vi "UMLEditor ScriptTaskUpdateDiagram.vi"(0 "Folder/LLB-Path":path, 1 "AggregateClassPaths":path[](array[path]), 2 "BaseClass Folder/LLB-Path":path, 5 "error in (no error)":errorcluster, 6 "AggregateClassNames":string[](array[string])) -> (19 "error out":errorcluster)   [LabVIEW 2016]
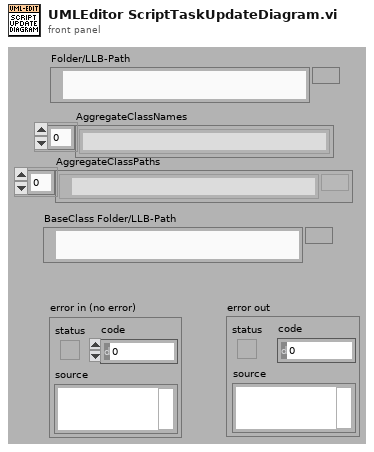
[diagram p1: front panel]
types:
  T1 = cluster{"CreateRef":refnum<vi>, "CreatePath":path, "CreateDiagram":refnum<vi>, "CalledCreatePaths":path[], "AggCreatePaths":path[], "DestroyRef":refnum<vi>, "DestroyPath":path, "DestroyDiagram":refnum<vi>, "CalledDestroyPaths":path[], "AggDestroyPaths":path[]}
  T2 = enum16{"NormalSubVis", "LV-Internal VIs", "All VIs", "All Functions"}
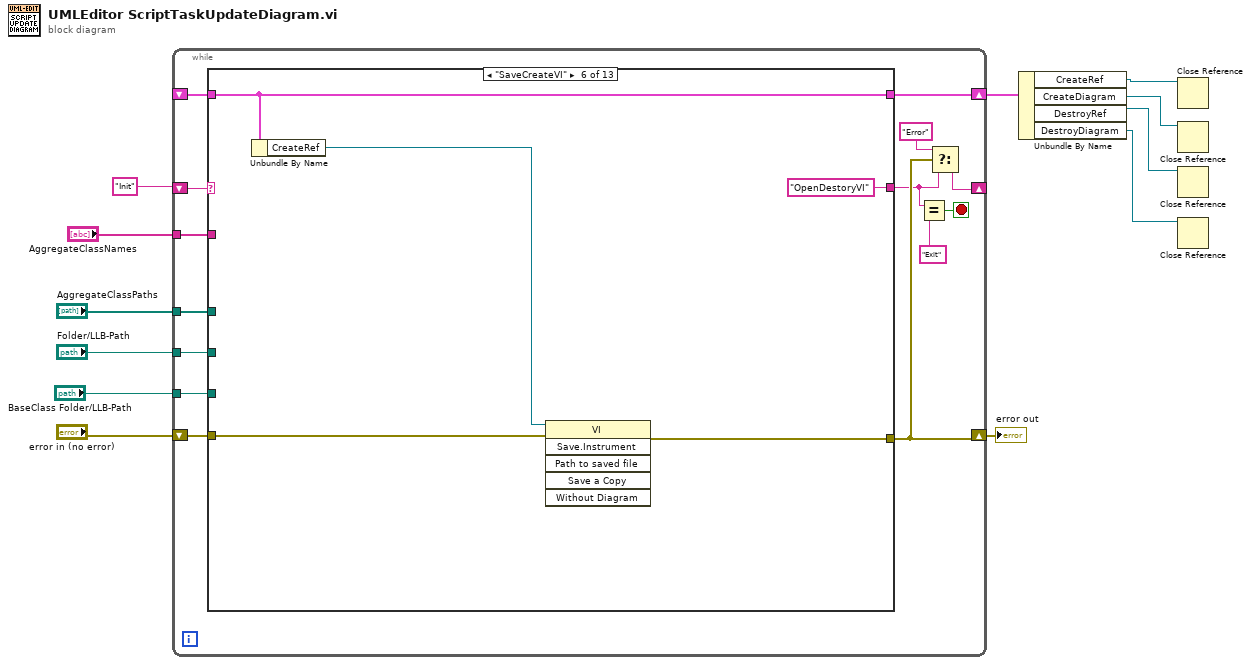
[diagram p0: block diagram]
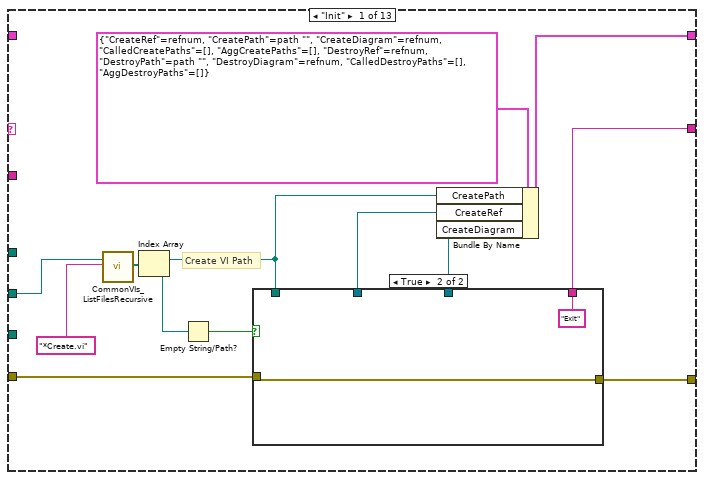
[diagram p2: hidden frame]
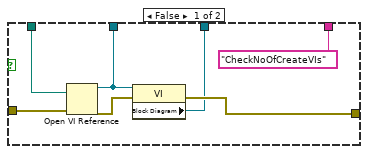
[diagram p3: hidden frame]
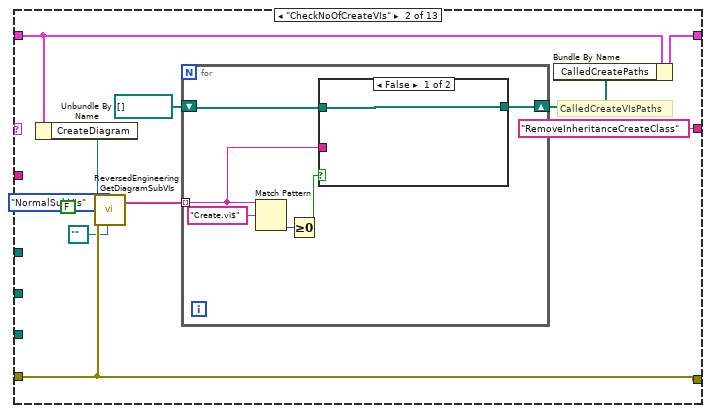
[diagram p4: hidden frame]
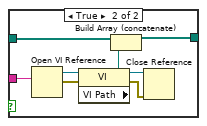
[diagram p5: hidden frame]
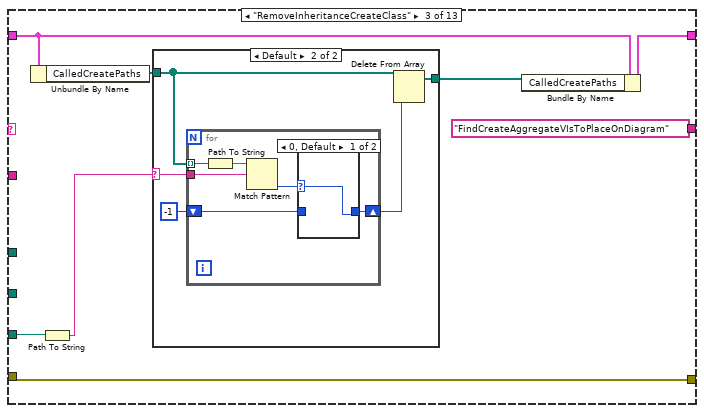
[diagram p6: hidden frame]
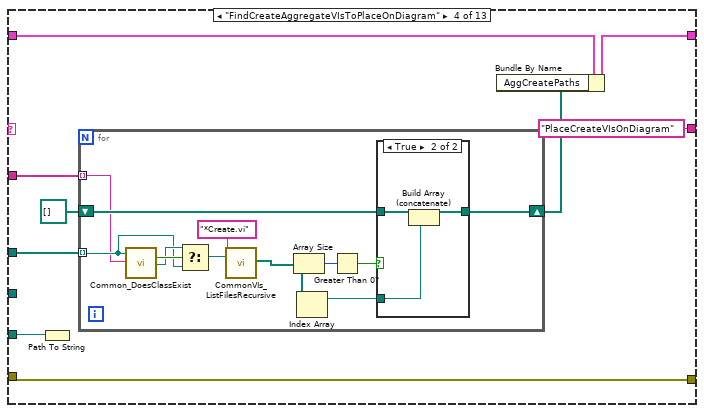
[diagram p9: hidden frame]
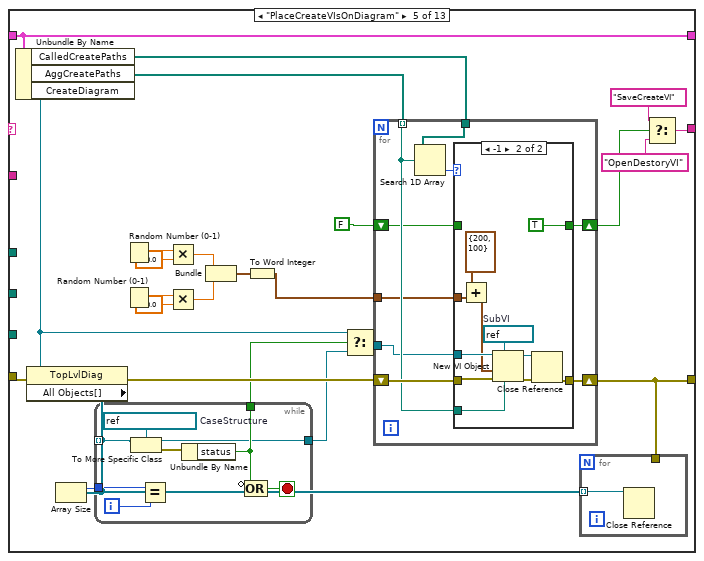
[diagram p11: hidden frame]
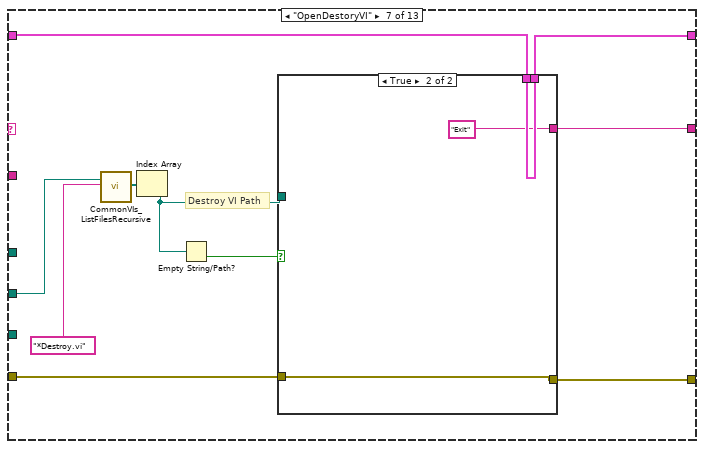
[diagram p13: hidden frame]
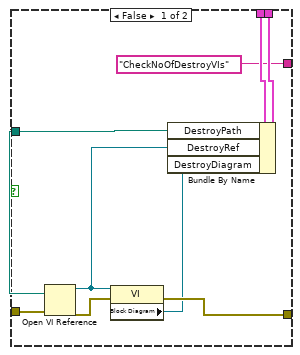
[diagram p14: hidden frame]
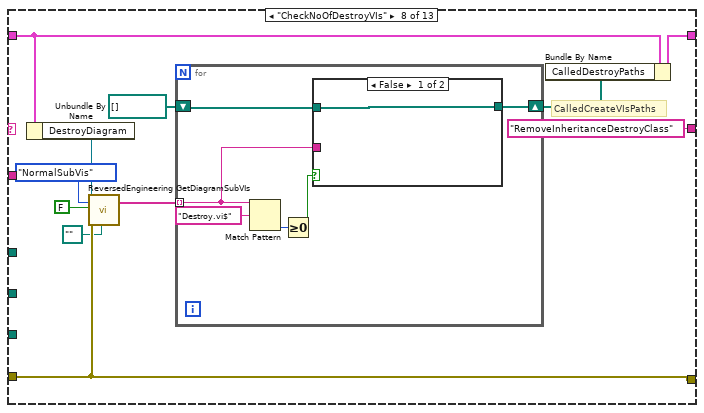
[diagram p15: hidden frame]
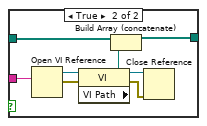
[diagram p16: hidden frame]
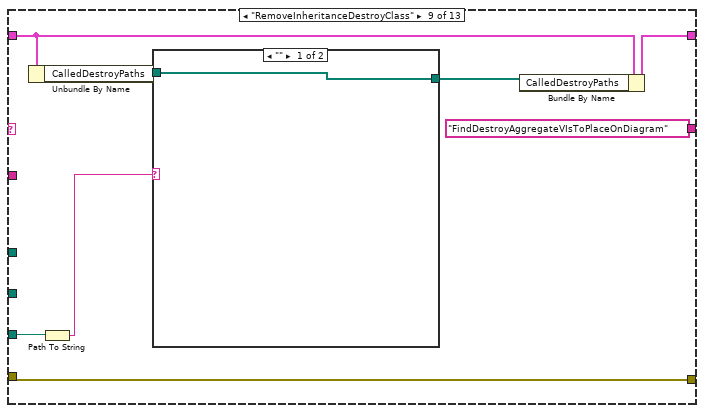
[diagram p17: hidden frame]
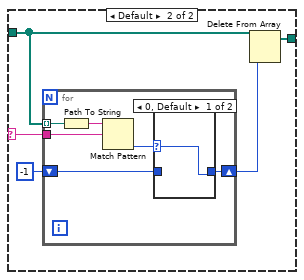
[diagram p18: hidden frame]
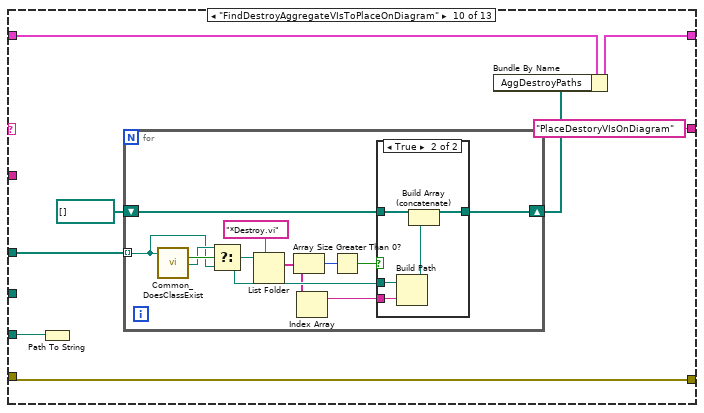
[diagram p20: hidden frame]
diagram:
  n1 = while {
    shift-right: [w23] -> _
    shift-left: "Init" -> [w26]
    shift-right: [w24] -> w9
    shift-left: "error in (no error)" -> [w25]
    shift-right: [w18] -> w11
    shift-left: _ -> [w17]
    tunnel: "Folder/LLB-Path" -> [w16]
    tunnel: "BaseClass Folder/LLB-Path" -> [w15]
    tunnel: "AggregateClassPaths" -> [w14]
    tunnel: "AggregateClassNames" -> [w13]
    stop <- w19 stop-if-true
    n2 = case shown="\"SaveCreateVI\"" w26 {
      selector: w26 -> [_ _ _ _ _ _ _ _ _ _ _ _ w340]
      tunnel: w25 -> [w38 w51 w76 w101 w141 w180 w191 w207 w232 w256 w297 w336 w339]
      tunnel: [w34 w51 w76 w101 w129 w178 w189 w207 w232 w256 w285 w334 w339] -> w24
      tunnel: [w27 "RemoveInheritanceCreateClass" "FindCreateAggregateVIsToPlaceOnDiagram" "PlaceCreateVIsOnDiagram" w133 "OpenDestoryVI" w182 "RemoveInheritanceDestroyClass" "FindDestroyAggregateVIsToPlaceOnDiagram" "PlaceDestoryVIsOnDiagram" w289 "Exit" "Exit"] -> w21
      tunnel: [w36 w54 w80 w103 w144 w177 w190 w210 w236 w258 w300 w333 w341] -> w18
      tunnel: w17 -> [_ w55 w81 w104 w144 w177 w188 w211 w237 w259 w300 w333 w341]
      tunnel: w16 -> [w32 _ _ _ _ _ w186 _ _ _ _ _ _]
      tunnel: w15 -> [_ _ w79 w102 _ _ _ _ w235 w257 _ _ _]
      tunnel: w14 -> [_ _ _ w99 _ _ _ _ _ w254 _ _ _]
      tunnel: w13 -> [_ _ _ w96 _ _ _ _ _ _ _ _ _]
      frame "Init" {
        # "Create VI Path"
        n3 = call <resource>:"CommonVIs_ListFilesRecursive.vi"("directory path"=w32, "FileSearchPattern"="*Create.vi" ("pattern")) -> ("Files"=w30:path[])  [unwired: 4 in, 13 out]
        n4 = Index Array(array=w30) -> (element=w29:path)  [unwired: 1 in]
        n5 = Empty String/Path?(string/path=w29) -> (empty?=w28:bool)
        n6 = case shown="True" w28 {
          tunnel: w38 -> [w45 w47]
          tunnel: w29 -> [w44 _]
          tunnel: [w43 _] -> w35
          tunnel: [w41 w47] -> w34
          tunnel: [w40 _] -> w33
          tunnel: ["CheckNoOfCreateVIs" "Exit"] -> w27
          frame False {
            n7 = Open VI Reference(vi path=w44, error in (no error)=w45) -> (vi reference=w43:refnum<vi>, error out=w42:errorcluster)  [unwired: 4 out]
            n8 = property class="VI"(reference=w43, error in=w42) -> (error out=w41:errorcluster, "Block Diagram"=w40:refnum<vi>)  [unwired: 1 out]
          }
          frame True {
          }
        }
        n9 = Bundle By Name(cluster=T1 {"CreateRef"=refnum, "CreatePath"=path "", "CreateDiagram"=refnum, "CalledCreatePaths"=[], "AggCreatePaths"=[], "DestroyRef"=refnum, "DestroyPath"=path "", "DestroyDiagram"=refnum, "CalledDestroyPaths"=[], "AggDestroyPaths"=[]}, "CreatePath"=w29, "CreateRef"=w35, "CreateDiagram"=w33) -> (w36:T1)
      }
      frame "CheckNoOfCreateVIs" {
        # "CalledCreateVIsPaths"
        n10 = Unbundle By Name(w55) -> ("CreateDiagram"=w58:refnum<vi>)
        n11 = call <resource>:"ReversedEngineering GetDiagramSubVIs.vi"("Diagram"=w58, "SubVIsOptions(NormalSubVis)"=T2."NormalSubVis", "RecrsiveSearchInNormalSubVIs(False)"=FALSE, "error in (no error)"=w51, "PathToDebugVI(OnlyUsedForRecursivVitFiles)"=path "") -> ("SubViNames"=w57:string[])  [unwired: 14 out]
        n12 = for {
          tunnel: w57 -> [w59] mode=indexing
          shift-right: [w61] -> w53
          shift-left: path[] [] -> [w62]
          n13 = Match Pattern(string=w59, regular expression="Create.vi$") -> (offset past match=w63:i32)  [unwired: 4 out]
          n14 = Greater Or Equal To 0?(x=w63) -> (x >= 0?=w60:bool)
          n15 = case shown="False" w60 {
            tunnel: w62 -> [w65 w73]
            tunnel: [w65 w69] -> w61
            tunnel: w59 -> [_ w72]
            frame False {
            }
            frame True {
              n16 = Open VI Reference(vi path=w72) -> (vi reference=w70:refnum<vi>, error out=w71:errorcluster)  [unwired: 1 in, 4 out]
              n17 = property class="VI"(reference=w70, error in=w71) -> (reference out=w67:refnum<vi>, error out=w66:errorcluster, "VI Path"=w68:path)
              n18 = Build Array (concatenate)(w73, w68) -> (w69:path[])
              n19 = Close Reference(reference=w67, error in (no error)=w66) -> ()  [unwired: 1 out]
            }
          }
        }
        n20 = Bundle By Name(cluster=w55, "CalledCreatePaths"=w53) -> (w54:T1)
      }
      frame "RemoveInheritanceCreateClass" {
        n21 = Unbundle By Name(w81) -> ("CalledCreatePaths"=w78:path[])
        n22 = Path To String(path=w79) -> (string=w74:string)
        n23 = case shown="Default" w74 {
          selector: w74 -> [_ w83]
          tunnel: w78 -> [w82 w86]
          tunnel: [w82 w85] -> w77
          frame "" {
          }
          frame Default {
            n24 = for {
              tunnel: w86 -> [w93] mode=indexing
              tunnel: w83 -> [w92]
              shift-right: [w89] -> w84
              shift-left: -1 ("offset past match") -> [w90]
              n25 = Path To String(path=w93) -> (string=w88:string)
              n26 = Match Pattern(string=w88, regular expression=w92) -> (offset past match=w91:i32)  [unwired: 4 out]
              n27 = case shown="0, Default" w91 {
                selector: w91 -> [w94 _]
                tunnel: w90 -> [_ w95]
                tunnel: [w94 w95] -> w89
                frame 0, Default {
                }
                frame -1 {
                }
              }
            }
            n28 = Delete From Array(array=w86, index=w84) -> (array with subset deleted=w85:path[])  [unwired: 1 in, 1 out]
          }
        }
        n29 = Bundle By Name(cluster=w81, "CalledCreatePaths"=w77) -> (w80:T1)
      }
      frame "FindCreateAggregateVIsToPlaceOnDiagram" {
        n30 = Path To String(path=w102) -> ()  [unwired: 1 out]
        n31 = for {
          shift-right: [w115] -> w97
          shift-left: path[] [] -> [w116]
          tunnel: w99 -> [w112] mode=indexing
          tunnel: w96 -> [w108] mode=indexing
          n32 = call <resource>:"Common_DoesClassExist.vi"("ClassPath"=w112, "ClassName"=w108) -> ("llb-class"=w114:bool, "llb/LvCLass-Path"=w113:path)  [unwired: 16 out]
          n33 = Select(t=w113, s=w114, f=w112) -> (s? t:f=w105:path)
          n34 = call <resource>:"CommonVIs_ListFilesRecursive.vi"("directory path"=w105, "FileSearchPattern"="*Create.vi" ("pattern")) -> ("Files"=w107:path[])  [unwired: 4 in, 13 out]
          n35 = Array Size(array=w107) -> (size(s)=w111:i32)
          n36 = Index Array(array=w107) -> (element=w109:path)  [unwired: 1 in]
          n37 = Greater Than 0?(x=w111) -> (x > 0?=w110:bool)
          n38 = case shown="True" w110 {
            tunnel: w116 -> [w117 w120]
            tunnel: [w117 w119] -> w115
            tunnel: w109 -> [_ w118]
            frame False {
            }
            frame True {
              n39 = Build Array (concatenate)(w120, w118) -> (w119:path[])
            }
          }
        }
        n40 = Bundle By Name(cluster=w104, "AggCreatePaths"=w97) -> (w103:T1)
      }
      frame "PlaceCreateVIsOnDiagram" {
        n41 = Unbundle By Name(w144) -> ("CalledCreatePaths"=w142:path[], "AggCreatePaths"=w143:path[], "CreateDiagram"=w137:refnum<vi>)
        n42 = property class="TopLvlDiag"(reference=w137, error in=w141) -> ("All Objects[]"=w131:refnum<vi>[])  [unwired: 2 out]
        n43 = Array Size(array=w131) -> (size(s)=w139:i32)
        n44 = while {
          tunnel: w131 -> [w154] mode=indexing
          tunnel: [w146] -> w130
          tunnel: w139 -> [w153]
          tunnel: [w148] -> w138
          i -> [w147]
          stop <- w150 stop-if-true
          w149 = refnum<vi> refnum  # CaseStructure
          n45 = To More Specific Class(target class=w149, reference=w154) -> (specific class reference=w146:refnum<vi>, error out=w151:errorcluster)  [unwired: 1 in]
          n46 = Equal?(x=w153, y=w147) -> (x = y?=w152:bool)
          n47 = Unbundle By Name(w151) -> ("status"=w148:bool)
          n48 = Compound Arithmetic op=OR(invert w148, w152) -> (w150:bool)
        }
        n49 = Random Number (0-1)() -> (number: 0 to 1=w128:dbl)
        n50 = Random Number (0-1)() -> (number: 0 to 1=w125:dbl)
        n51 = Multiply(x=w128, y=100.0) -> (x*y=w124:dbl)
        n52 = Multiply(x=w125, y=100.0) -> (x*y=w123:dbl)
        n53 = Bundle(w124, w123) -> (w122:cluster{dbl, dbl})  [unwired: 1 out]
        n54 = To Word Integer(number=w122) -> (16bit integer=w121:cluster{i16, i16})
        n55 = Select(t=w137, s=w138, f=w130) -> (s? t:f=w140:refnum<vi>)
        n56 = for {
          shift-right: [w160] -> w129
          shift-left: w141 -> [w161]
          tunnel: w143 -> [w159] mode=indexing
          tunnel: w142 -> [w163]
          tunnel: w140 -> [w158]
          shift-right: [w157] -> w135
          shift-left: FALSE -> [w156]
          tunnel: w121 -> [w155]
          n57 = Search 1D Array(1D array=w163, element=w159) -> (index of element=w162:i32)  [unwired: 1 out]
          n58 = case shown="-1" w162 {
            tunnel: w161 -> [w165 w175]
            tunnel: [w165 w169] -> w160
            tunnel: w158 -> [_ w176]
            tunnel: w159 -> [_ w172]
            tunnel: [w164 TRUE] -> w157
            tunnel: w156 -> [w164 _]
            tunnel: w155 -> [_ w166]
            frame 0, Default {
            }
            frame -1 {
              w173 = refnum<vi> refnum  # SubVI
              n59 = Add(x=cluster{"Horizontal":i16, "Vertical":i16} {"Horizontal"=200, "Vertical"=100} ("position/next to"), y=w166) -> (x+y=w167:cluster{i16, i16})
              n60 = New VI Object(vi object class=w173, owner refnum=w176, position/next to=w167, 6:w172, 8:w175) -> (object refnum=w168:refnum<vi>, 0:w170:errorcluster)  [unwired: 3 out]
              n61 = Close Reference(reference=w168, error in (no error)=w170) -> (error out=w169:errorcluster)
            }
          }
        }
        n62 = for {
          tunnel: w131 -> [w145] mode=indexing
          tunnel: w129 -> [_]
          n63 = Close Reference(reference=w145) -> ()  [unwired: 1 in, 1 out]
        }
        n64 = Select(t="SaveCreateVI", s=w135, f="OpenDestoryVI") -> (s? t:f=w133:string)
      }
      frame "SaveCreateVI" {
        n65 = Unbundle By Name(w177) -> ("CreateRef"=w179:refnum<vi>)
        n66 = invoke class="VI" method="Save.Instrument"(reference=w179, error in=w180) -> (error out=w178:errorcluster)  [unwired: 4 in, 5 out]
      }
      frame "OpenDestoryVI" {
        # "Destroy VI Path"
        n67 = call <resource>:"CommonVIs_ListFilesRecursive.vi"("directory path"=w186, "FileSearchPattern"="*Destroy.vi" ("pattern")) -> ("Files"=w187:path[])  [unwired: 4 in, 13 out]
        n68 = Index Array(array=w187) -> (element=w184:path)  [unwired: 1 in]
        n69 = Empty String/Path?(string/path=w184) -> (empty?=w183:bool)
        n70 = case shown="True" w183 {
          tunnel: w191 -> [w200 w201]
          tunnel: [w199 w203] -> w190
          tunnel: [w196 w201] -> w189
          tunnel: w188 -> [w194 w203]
          tunnel: w184 -> [w193 _]
          tunnel: ["CheckNoOfDestroyVIs" "Exit"] -> w182
          frame False {
            n71 = Open VI Reference(vi path=w193, error in (no error)=w200) -> (vi reference=w198:refnum<vi>, error out=w197:errorcluster)  [unwired: 4 out]
            n72 = property class="VI"(reference=w198, error in=w197) -> (error out=w196:errorcluster, "Block Diagram"=w195:refnum<vi>)  [unwired: 1 out]
            n73 = Bundle By Name(cluster=w194, "DestroyPath"=w193, "DestroyRef"=w198, "DestroyDiagram"=w195) -> (w199:T1)
          }
          frame True {
          }
        }
      }
      frame "CheckNoOfDestroyVIs" {
        # "CalledCreateVIsPaths"
        n74 = Unbundle By Name(w211) -> ("DestroyDiagram"=w214:refnum<vi>)
        n75 = call <resource>:"ReversedEngineering GetDiagramSubVIs.vi"("Diagram"=w214, "SubVIsOptions(NormalSubVis)"=T2."NormalSubVis", "RecrsiveSearchInNormalSubVIs(False)"=FALSE, "error in (no error)"=w207, "PathToDebugVI(OnlyUsedForRecursivVitFiles)"=path "") -> ("SubViNames"=w213:string[])  [unwired: 14 out]
        n76 = for {
          tunnel: w213 -> [w215] mode=indexing
          shift-right: [w217] -> w209
          shift-left: path[] [] -> [w218]
          n77 = Match Pattern(string=w215, regular expression="Destroy.vi$") -> (offset past match=w219:i32)  [unwired: 4 out]
          n78 = Greater Or Equal To 0?(x=w219) -> (x >= 0?=w216:bool)
          n79 = case shown="False" w216 {
            tunnel: w218 -> [w221 w229]
            tunnel: [w221 w225] -> w217
            tunnel: w215 -> [_ w228]
            frame False {
            }
            frame True {
              n80 = Open VI Reference(vi path=w228) -> (vi reference=w226:refnum<vi>, error out=w227:errorcluster)  [unwired: 1 in, 4 out]
              n81 = property class="VI"(reference=w226, error in=w227) -> (reference out=w223:refnum<vi>, error out=w222:errorcluster, "VI Path"=w224:path)
              n82 = Build Array (concatenate)(w229, w224) -> (w225:path[])
              n83 = Close Reference(reference=w223, error in (no error)=w222) -> ()  [unwired: 1 out]
            }
          }
        }
        n84 = Bundle By Name(cluster=w211, "CalledDestroyPaths"=w209) -> (w210:T1)
      }
      frame "RemoveInheritanceDestroyClass" {
        n85 = Unbundle By Name(w237) -> ("CalledDestroyPaths"=w234:path[])
        n86 = Path To String(path=w235) -> (string=w230:string)
        n87 = case shown="\"\"" w230 {
          selector: w230 -> [_ w239]
          tunnel: w234 -> [w238 w242]
          tunnel: [w238 w241] -> w233
          frame "" {
          }
          frame Default {
            n88 = for {
              tunnel: w242 -> [w249] mode=indexing
              tunnel: w239 -> [w248]
              shift-right: [w245] -> w240
              shift-left: -1 ("offset past match") -> [w246]
              n89 = Path To String(path=w249) -> (string=w244:string)
              n90 = Match Pattern(string=w244, regular expression=w248) -> (offset past match=w247:i32)  [unwired: 4 out]
              n91 = case shown="0, Default" w247 {
                selector: w247 -> [w250 _]
                tunnel: w246 -> [_ w251]
                tunnel: [w250 w251] -> w245
                frame 0, Default {
                }
                frame -1 {
                }
              }
            }
            n92 = Delete From Array(array=w242, index=w240) -> (array with subset deleted=w241:path[])  [unwired: 1 in, 1 out]
          }
        }
        n93 = Bundle By Name(cluster=w237, "CalledDestroyPaths"=w233) -> (w236:T1)
      }
      frame "FindDestroyAggregateVIsToPlaceOnDiagram" {
        n94 = Path To String(path=w257) -> ()  [unwired: 1 out]
        n95 = for {
          shift-right: [w269] -> w252
          shift-left: path[] [] -> [w270]
          tunnel: w254 -> [w266] mode=indexing
          n96 = call <resource>:"Common_DoesClassExist.vi"("ClassPath"=w266) -> ("llb-class"=w268:bool, "llb/LvCLass-Path"=w267:path)  [unwired: 1 in, 16 out]
          n97 = Select(t=w267, s=w268, f=w266) -> (s? t:f=w262:path)
          n98 = List Folder(path=w262, pattern="*Destroy.vi") -> (filenames=w261:string[])  [unwired: 1 in, 4 out]
          n99 = Array Size(array=w261) -> (size(s)=w264:i32)
          n100 = Index Array(array=w261) -> (element=w260:string)  [unwired: 1 in]
          n101 = Greater Than 0?(x=w264) -> (x > 0?=w263:bool)
          n102 = case shown="True" w263 {
            tunnel: w270 -> [w271 w276]
            tunnel: [w271 w275] -> w269
            tunnel: w262 -> [_ w274]
            tunnel: w260 -> [_ w273]
            frame False {
            }
            frame True {
              n103 = Build Path(base path=w274, name or relative path=w273) -> (appended path=w272:path)
              n104 = Build Array (concatenate)(w276, w272) -> (w275:path[])
            }
          }
        }
        n105 = Bundle By Name(cluster=w259, "AggDestroyPaths"=w252) -> (w258:T1)
      }
      frame "PlaceDestoryVIsOnDiagram" {
        n106 = Unbundle By Name(w300) -> ("CalledDestroyPaths"=w298:path[], "AggDestroyPaths"=w299:path[], "DestroyDiagram"=w293:refnum<vi>)
        n107 = property class="TopLvlDiag"(reference=w293, error in=w297) -> ("All Objects[]"=w287:refnum<vi>[])  [unwired: 2 out]
        n108 = Array Size(array=w287) -> (size(s)=w295:i32)
        n109 = while {
          tunnel: w287 -> [w310] mode=indexing
          tunnel: [w302] -> w286
          tunnel: w295 -> [w309]
          tunnel: [w304] -> w294
          i -> [w303]
          stop <- w306 stop-if-true
          w305 = refnum<vi> refnum  # CaseStructure
          n110 = To More Specific Class(target class=w305, reference=w310) -> (specific class reference=w302:refnum<vi>, error out=w307:errorcluster)  [unwired: 1 in]
          n111 = Equal?(x=w309, y=w303) -> (x = y?=w308:bool)
          n112 = Unbundle By Name(w307) -> ("status"=w304:bool)
          n113 = Compound Arithmetic op=OR(invert w304, w308) -> (w306:bool)
        }
        n114 = Random Number (0-1)() -> (number: 0 to 1=w284:dbl)
        n115 = Random Number (0-1)() -> (number: 0 to 1=w281:dbl)
        n116 = Multiply(x=w284, y=100.0) -> (x*y=w280:dbl)
        n117 = Multiply(x=w281, y=100.0) -> (x*y=w279:dbl)
        n118 = Bundle(w280, w279) -> (w278:cluster{dbl, dbl})  [unwired: 1 out]
        n119 = To Word Integer(number=w278) -> (16bit integer=w277:cluster{i16, i16})
        n120 = Select(t=w293, s=w294, f=w286) -> (s? t:f=w296:refnum<vi>)
        n121 = for {
          shift-right: [w316] -> w285
          shift-left: w297 -> [w317]
          tunnel: w299 -> [w315] mode=indexing
          tunnel: w298 -> [w319]
          tunnel: w296 -> [w314]
          shift-right: [w313] -> w291
          shift-left: FALSE -> [w312]
          tunnel: w277 -> [w311]
          n122 = Search 1D Array(1D array=w319, element=w315) -> (index of element=w318:i32)  [unwired: 1 out]
          n123 = case shown="-1" w318 {
            tunnel: w317 -> [w321 w331]
            tunnel: [w321 w326] -> w316
            tunnel: w314 -> [_ w332]
            tunnel: w315 -> [_ w329]
            tunnel: [w320 TRUE] -> w313
            tunnel: w312 -> [w320 _]
            tunnel: w311 -> [_ w324]
            frame 0, Default {
            }
            frame -1 {
              w330 = refnum<vi> refnum  # SubVI
              n124 = Add(x=cluster{"Horizontal":i16, "Vertical":i16} {"Horizontal"=100, "Vertical"=100} ("position/next to"), y=w324) -> (x+y=w322:cluster{i16, i16})
              n125 = New VI Object(vi object class=w330, owner refnum=w332, position/next to=w322, 6:w329, 8:w331) -> (object refnum=w325:refnum<vi>, 0:w327:errorcluster)  [unwired: 3 out]
              n126 = Close Reference(reference=w325, error in (no error)=w327) -> (error out=w326:errorcluster)
            }
          }
        }
        n127 = for {
          tunnel: w287 -> [w301] mode=indexing
          tunnel: w285 -> [_]
          n128 = Close Reference(reference=w301) -> ()  [unwired: 1 in, 1 out]
        }
        n129 = Select(t="SaveDestroyVI", s=w291, f="Exit") -> (s? t:f=w289:string)
      }
      frame "SaveDestroyVI" {
        n130 = Unbundle By Name(w333) -> ("DestroyRef"=w335:refnum<vi>)
        n131 = invoke class="VI" method="Save.Instrument"(reference=w335, error in=w336) -> (error out=w334:errorcluster)  [unwired: 4 in, 5 out]
      }
      frame "Error", Default {
        n132 = Unbundle By Name(w339) -> ("source"=w338:string)
        n133 = One Button Dialog(message=w338, button name ("OK")=w340) -> ()  [unwired: 1 out]
      }
    }
    n134 = Equal?(x=w21, y="Exit") -> (x = y?=w19:bool)
    n135 = Select(t="Error", s=w24, f=w21) -> (s? t:f=w23:string)
  }
  "error out" <- w9
  n136 = Unbundle By Name(w11) -> ("CreateRef"=w10:refnum<vi>, "CreateDiagram"=w4:refnum<vi>, "DestroyRef"=w3:refnum<vi>, "DestroyDiagram"=w2:refnum<vi>)
  n137 = Close Reference(reference=w10) -> ()  [unwired: 1 in, 1 out]
  n138 = Close Reference(reference=w4) -> ()  [unwired: 1 in, 1 out]
  n139 = Close Reference(reference=w3) -> ()  [unwired: 1 in, 1 out]
  n140 = Close Reference(reference=w2) -> ()  [unwired: 1 in, 1 out]
